vi "Update State Data.vi"(8 "error in (no error)":errorcluster, 9 "Data":variant, 10 "Argument":string, 11 "Image Assertion in":refnum<class "Image Assertion.lvclass">) -> (0 "error out":errorcluster, 3 "Image Assertion out":refnum<class "Image Assertion.lvclass">)   [LabVIEW 2020, in "MacroAssert.lvlib" / "Image Assertion.lvclass"]
uses:
  Image Assertion.lvclass
  Image Assertion Type.ctl
  Image Comparator.ctl
  Assertion Step/Assertion Step.lvclass
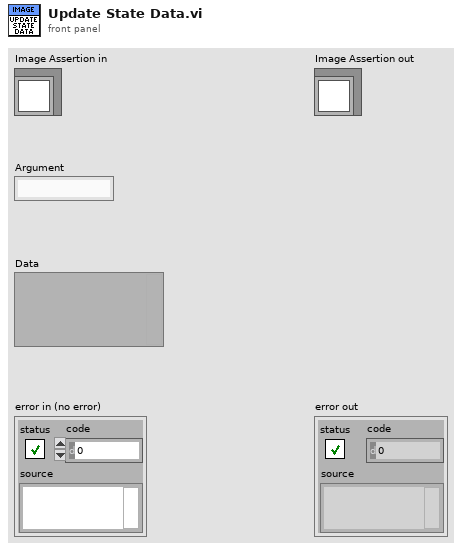
[diagram p1: front panel]
types:
  T1 = typedef "MacroAssert.lvlib/Image Assertion.lvclass/Image Assertion Type.ctl" = enum16{"Control Image", "VI Image", "Window Image"}
  T2 = typedef "MacroAssert.lvlib/Image Assertion.lvclass/Image Comparator.ctl" = enum16{"Equals", "Does not equal"}
  T3 = typedef "imagedata.ctl" = cluster{"image type":i32, "image depth":i32, "image":u8[], "mask":u8[], "colors":u32[], "Rectangle":cluster{"left":i16, "top":i16, "right":i16, "bottom":i16}}
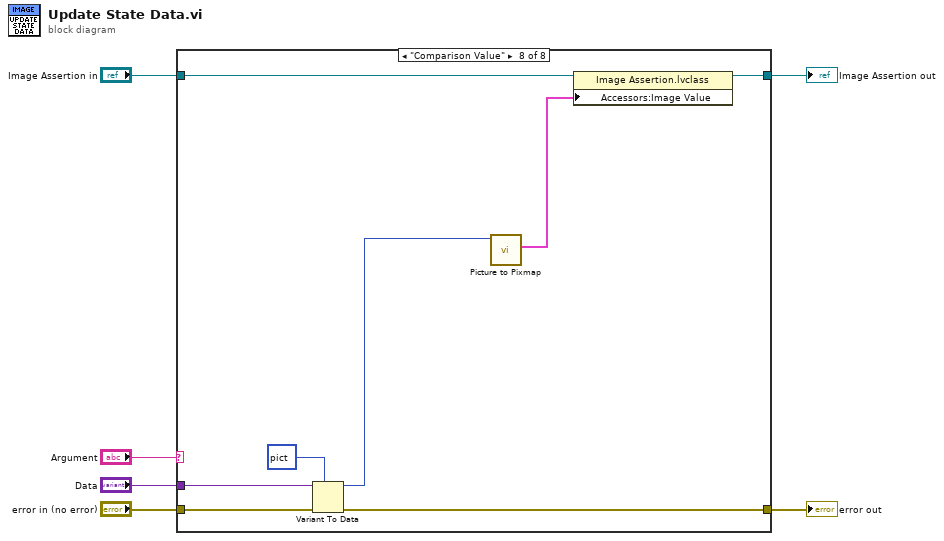
[diagram p0: block diagram]
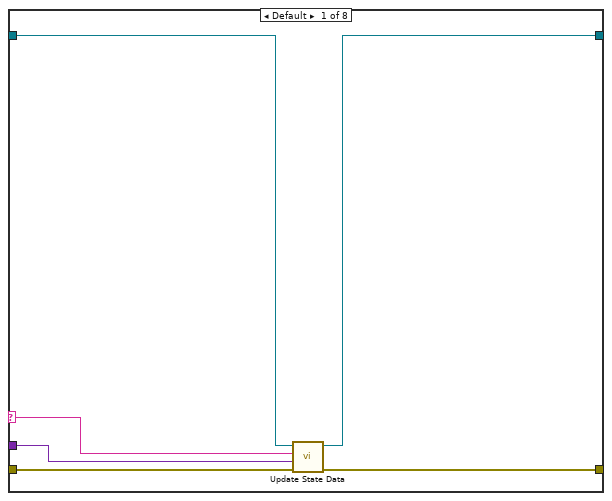
[diagram p2: hidden frame]
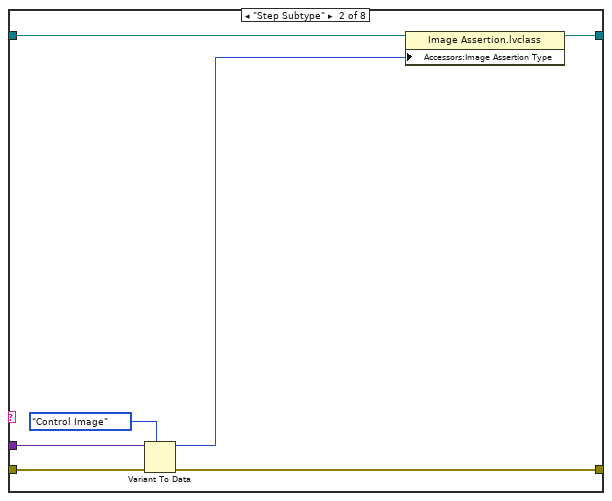
[diagram p3: hidden frame]
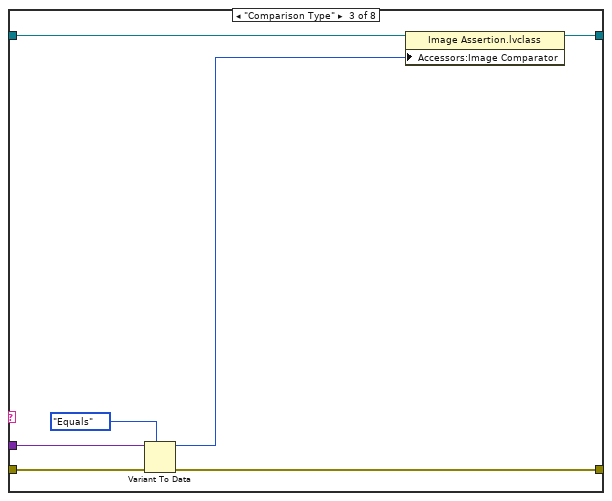
[diagram p4: hidden frame]
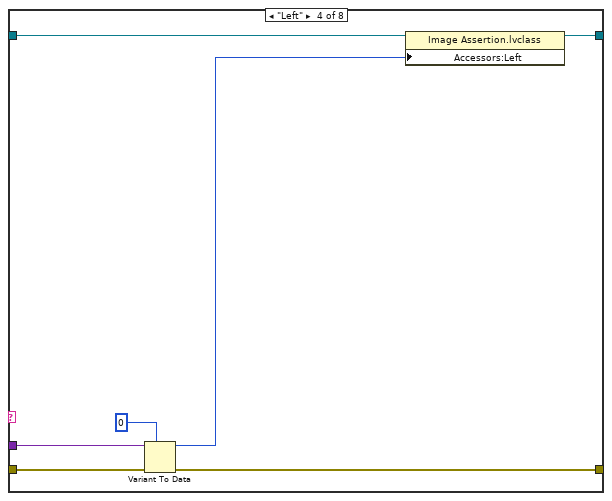
[diagram p5: hidden frame]
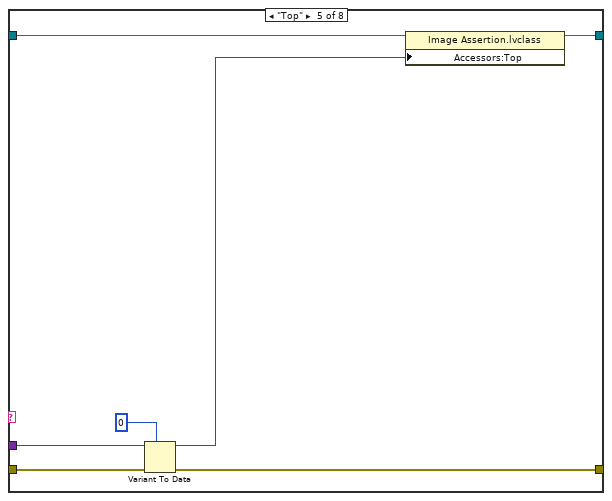
[diagram p6: hidden frame]
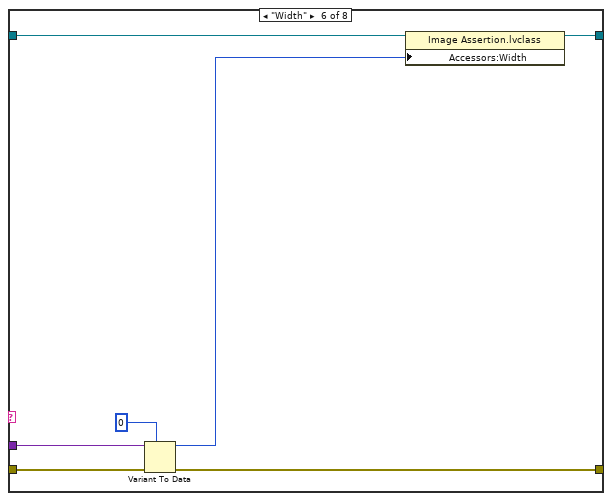
[diagram p7: hidden frame]
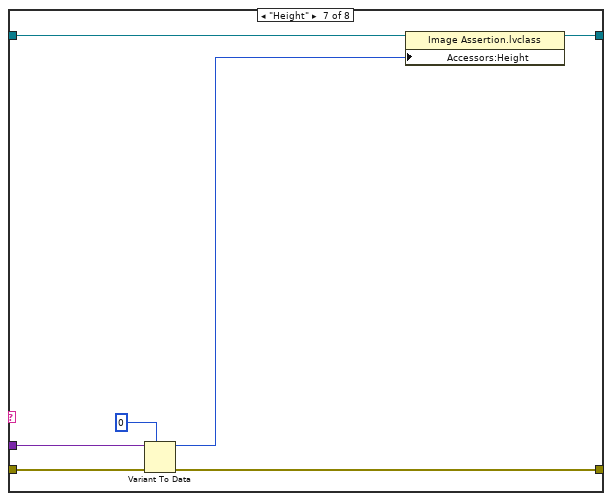
[diagram p8: hidden frame]
diagram:
  n1 = case shown="\"Comparison Value\"" "Argument" {
    selector: "Argument" -> [w7 _ _ _ _ _ _ _]
    tunnel: "Image Assertion in" -> [w10 w19 w26 w33 w40 w47 w54 w62]
    tunnel: "error in (no error)" -> [w12 w17 w24 w31 w38 w45 w52 w60]
    tunnel: [w9 w18 w25 w32 w39 w46 w53 w61] -> w1
    tunnel: [w11 w16 w23 w30 w37 w44 w51 w59] -> w5
    tunnel: "Data" -> [w8 w15 w22 w29 w36 w43 w50 w58]
    frame Default {
      n2 = call-parent "Update State Data.vi"("error in (no error)"=w12, "Data"=w8, "Argument"=w7, "Assertion Step in"=w10) -> ("error out"=w11:errorcluster, "Assertion Step out"=w9:refnum<class "Image Assertion.lvclass">)  [unwired: 6 in]
    }
    frame "Step Subtype" {
      n3 = Variant To Data(error in=w17, type=Image_Assertion_Type."Control Image" ("NewVal"), Variant=w15) -> (data=w14:T1, error out=w16:errorcluster)
      n4 = property class="Image Assertion.lvclass"(reference=w19, "Accessors:Image Assertion Type"=w14) -> (reference out=w18:refnum<class "Image Assertion.lvclass">)  [unwired: 1 in, 1 out]
    }
    frame "Comparison Type" {
      n5 = Variant To Data(error in=w24, type=Image_Comparator."Equals" ("NewVal"), Variant=w22) -> (data=w21:T2, error out=w23:errorcluster)
      n6 = property class="Image Assertion.lvclass"(reference=w26, "Accessors:Image Comparator"=w21) -> (reference out=w25:refnum<class "Image Assertion.lvclass">)  [unwired: 1 in, 1 out]
    }
    frame "Left" {
      n7 = Variant To Data(error in=w31, type=i16 0, Variant=w29) -> (data=w28:i16, error out=w30:errorcluster)
      n8 = property class="Image Assertion.lvclass"(reference=w33, "Accessors:Left"=w28) -> (reference out=w32:refnum<class "Image Assertion.lvclass">)  [unwired: 1 in, 1 out]
    }
    frame "Top" {
      n9 = Variant To Data(error in=w38, type=i16 0, Variant=w36) -> (data=w35:i16, error out=w37:errorcluster)
      n10 = property class="Image Assertion.lvclass"(reference=w40, "Accessors:Top"=w35) -> (reference out=w39:refnum<class "Image Assertion.lvclass">)  [unwired: 1 in, 1 out]
    }
    frame "Width" {
      n11 = Variant To Data(error in=w45, type=i16 0, Variant=w43) -> (data=w42:i16, error out=w44:errorcluster)
      n12 = property class="Image Assertion.lvclass"(reference=w47, "Accessors:Width"=w42) -> (reference out=w46:refnum<class "Image Assertion.lvclass">)  [unwired: 1 in, 1 out]
    }
    frame "Height" {
      n13 = Variant To Data(error in=w52, type=i16 0, Variant=w50) -> (data=w49:i16, error out=w51:errorcluster)
      n14 = property class="Image Assertion.lvclass"(reference=w54, "Accessors:Height"=w49) -> (reference out=w53:refnum<class "Image Assertion.lvclass">)  [unwired: 1 in, 1 out]
    }
    frame "Comparison Value" {
      n15 = Variant To Data(error in=w60, type=picture data[5B] ("picture"), Variant=w58) -> (data=w56:picture, error out=w59:errorcluster)
      n16 = call <vilib>:"Picture to Pixmap.vi"("picture"=w56) -> ("image data"=w55:T3)  [unwired: 9 in, 1 out]
      n17 = property class="Image Assertion.lvclass"(reference=w62, "Accessors:Image Value"=w55) -> (reference out=w61:refnum<class "Image Assertion.lvclass">)  [unwired: 1 in, 1 out]
    }
  }
  "error out" <- w5
  "Image Assertion out" <- w1
